vi "Stop Core.vi"(10 "final error code":i32, 11 "CS++GoBangClient in":refnum<class "CS++GoBangClient.lvclass">) -> (3 "CS++GoBangClient out":refnum<class "CS++GoBangClient.lvclass">)   [LabVIEW 2014, in "GoBang.lvlib" / "CS++GoBangClient.lvclass"]
doc: "(<B>Filename</B>: Actor Framework.lvlib:Actor.lvclass:Stop Core.vi)\n\nDefines what the actor does before it stops. Use the <B>final error code</B> input to determine whether the actor shut down in response to an error.\n\nBy default, this method does nothing. A descendant class may override it to define behavior, such as shutting down any processes the actor initiated in its override of the Actor Core method."
uses:
  CS++GoBangClient.lvclass
  CS++GoBangClient.lvclass/CS++GoBangClient.ctl
  <vilib>/ActorFramework/Message Enqueuer/Message Enqueuer.lvclass/Message Enqueuer.ctl
  <vilib>/ActorFramework/Message Enqueuer/Enqueue.vi
  <vilib>/ActorFramework/Message Priority Queue/Priority Enqueue.vi
  <vilib>/ActorFramework/Stop Msg/Stop Msg.lvclass
  CSPP_Core/Actors/CS++BaseActor/CS++BaseActor.lvclass
  CSPP_Core/Classes/CS++ProcessVariables/PVConnection/PVConnection.lvclass
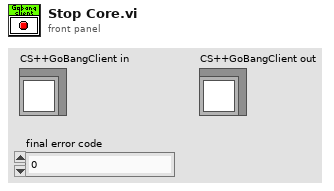
[diagram p1: front panel]
types:
  T1 = cluster{"JoinGame":refnum<class "PVConnection.lvclass">, "UpdateBoard":refnum<class "PVConnection.lvclass">}
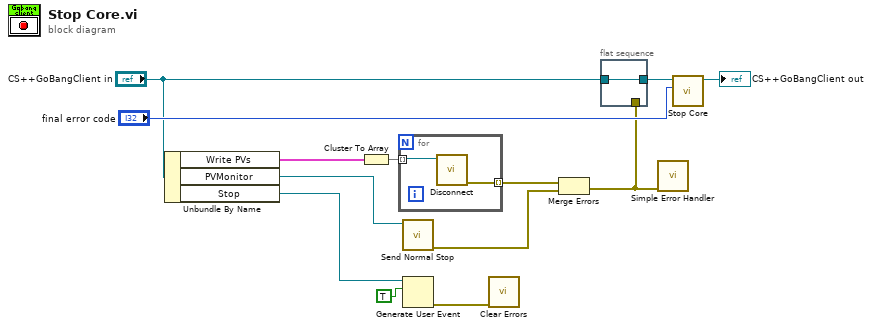
[diagram p0: block diagram]
diagram:
  n1 = Unbundle By Name("CS++GoBangClient in") -> ("Write PVs"=w11:T1, "PVMonitor"=w9:refnum<class "Message Enqueuer.lvclass">, "Stop"=w6:refnum<user-event>)
  n2 = Cluster To Array(cluster=w11) -> (array=w10:refnum<class "PVConnection.lvclass">[])
  n3 = for {
    tunnel: w10 -> [w15] mode=indexing
    tunnel: [w14] -> w8 mode=indexing
    n4 = call "Disconnect.vi"("PVConnection in"=w15) -> ("error out"=w14:errorcluster)  [unwired: 9 in, 1 out]
  }
  n5 = call <vilib>:"Send Normal Stop.vi"("Message Enqueuer"=w9) -> ("error out"=w7:errorcluster)  [unwired: 10 in]
  n6 = Generate User Event(user event=w6, event data cluster=TRUE ("event data")) -> (error out=w1:errorcluster)  [unwired: 2 in, 1 out]
  n7 = call <vilib>:"Clear Errors.vi"("error in (no error)"=w1) -> ()  [unwired: 5 in, 2 out]
  n8 = Merge Errors(w8, w7) -> (w2:errorcluster)
  n9 = flat-sequence {
    tunnel: "CS++GoBangClient in" -> [w16]
    tunnel: [w16] -> w3
    tunnel: w2 -> [_]
    frame #0 {
    }
  }
  n10 = call <vilib>:"Simple Error Handler.vi"("error in (no error)"=w2) -> ()  [unwired: 4 in, 5 out]
  n11 = call-parent "Stop Core.vi"("final error code"="final error code", "CS++BaseActor in"=w3) -> ("CS++BaseActor out"=→"CS++GoBangClient out":refnum<class "CS++GoBangClient.lvclass">)  [unwired: 9 in]
